vi "Unwrap angle (mod).vi"(11 "Numeric in":dbl[unit]) -> (3 "Numeric out":dbl[unit])   [LabVIEW 2019]
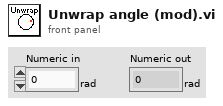
[diagram p1: front panel]
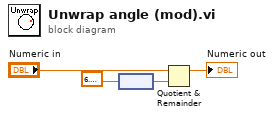
[diagram p0: block diagram]
diagram:
  n1 = node(6.283185307179586) -> (w3:dbl[unit])
  n2 = Quotient & Remainder(x="Numeric in", y=w3) -> (x-y*floor(x/y)=→"Numeric out":dbl[unit])  [unwired: 1 out]
